vi "Setup subWorker - ChartView.vi"(8 "error in":errorcluster, 11 "Manager Worker in":refnum<class "Manager Worker.lvclass">) -> (0 "error out":errorcluster, 3 "Manager Worker out":refnum<class "Manager Worker.lvclass">)   [LabVIEW 2018, in "Manager Worker.lvclass"]
doc: "<b>Note: Do not change the code in this VI!</b>\nThis VI performs a setup of all the statically-linked subWorkers that belong to the Worker that calls this VI. This VI is created automatically by the 'Create/Add Worker' tool and must be called <b>before</b> any statically linked subWorkers are called."
uses:
  Manager Worker.lvclass
  Manager Worker.lvclass/Manager Worker.ctl
  ChartView Worker/ChartView Worker.lvclass
  D:/Program Files (x86)/National Instruments/LabVIEW 2018/vi.lib/addons/_Workers/Library/Classes/Worker/Worker.lvclass
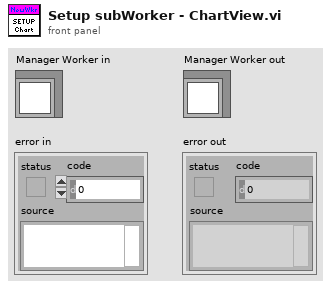
[diagram p1: front panel]
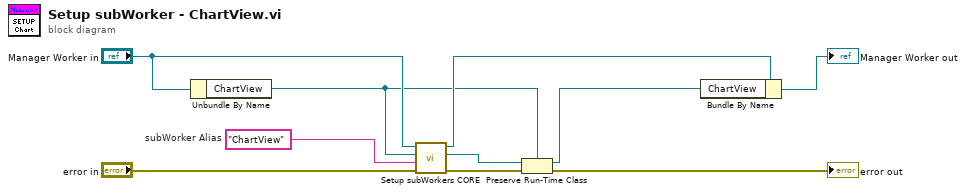
[diagram p0: block diagram]
diagram:
  w6 = "ChartView"  # subWorker Alias
  n1 = Unbundle By Name("Manager Worker in") -> ("ChartView"=w3:refnum<class "ChartView Worker.lvclass">)
  n2 = call-dynamic "Setup subWorkers CORE.vi"("error in"="error in", "subWorker Alias"=w6, "subWorker"=w3, "Worker"="Manager Worker in") -> ("error out"=w5:errorcluster, "subWorker out"=w1:refnum<class "Worker.lvclass">, "Worker out"=w8:refnum<class "Manager Worker.lvclass">)  [unwired: 5 in]
  n3 = Preserve Run-Time Class(object in=w1, error in=w5, 2:w3) -> (object out=w2:refnum<class "ChartView Worker.lvclass">, error out=→"error out":errorcluster)
  n4 = Bundle By Name(cluster=w8, "ChartView"=w2) -> (→"Manager Worker out":refnum<class "Manager Worker.lvclass">)
